vi "Get Exported Frames.vi"(8 "error in (no error)":errorcluster, 10 "GUID":string, 11 "Item Ref in":T4 format="%.0x") -> (0 "error out":errorcluster, 2 "Section":T1 {"Frames"."Signals"."Byte Order" items=["Little Endian", "Big Endian"]; "Frames"."Signals"."Data Type" items=["Signed", "Unsigned", "IEEE Float"]}, 3 "Section Ref out":T4 format="%.0x")   [LabVIEW 2015, in "Diagnostics Addon System Explorer.lvlib"]
uses:
  Diagnostics Addon System Explorer.lvlib
  <vilib>/NI Veristand/Custom Device Tools/Custom Device Utility Library/Custom Device Utility Library.lvlib
  <vilib>/NI Veristand/Custom Device Tools/Custom Device Utility Library/NI VeriStand - Search for Item by GUID.vi
  <vilib>/NI Veristand/Custom Device API/Custom Device API.lvlib
  Shared/Signal Parameters.ctl
  Shared/Diagnostics Addon Shared.lvlib
  Shared/Frame Parameters.ctl
  Shared/Exported Frames Cluster.ctl
  Shared/FG Action.ctl
  <vilib>/NI Veristand/Custom Device API/Custom Device Item Ref.ctl
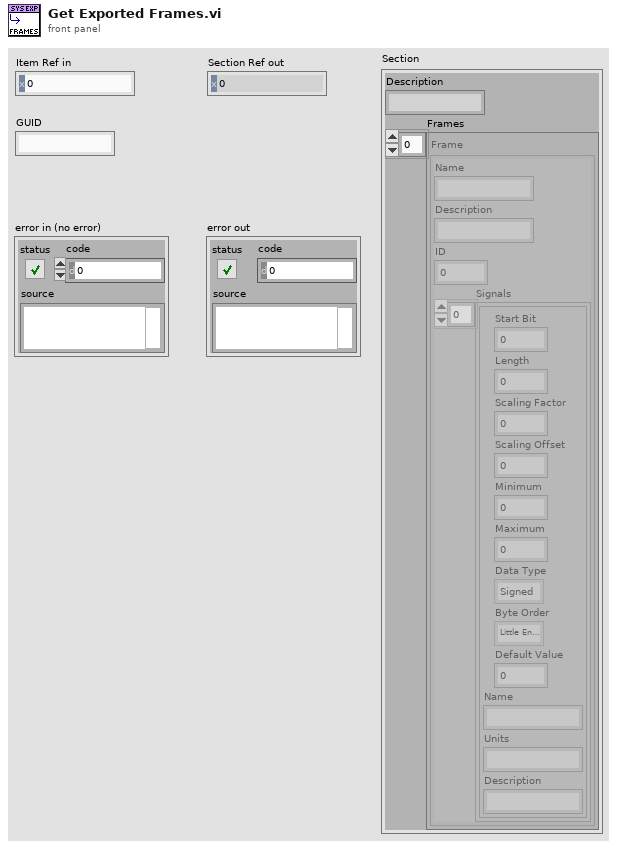
[diagram p1: front panel]
types:
  T1 = typedef "Diagnostics Addon System Explorer.lvlib/Exported Frames Cluster.ctl" = cluster{"Description":string, "Frames":T2[]}
  T2 = typedef "Diagnostics Addon Shared.lvlib/Frame Parameters.ctl" = cluster{"Name":string, "Description":string, "ID":u16, "Signals":T3[]}
  T3 = typedef "Diagnostics Addon Shared.lvlib/Signal Parameters.ctl" = cluster{"Start Bit":u8, "Length":u8, "Scaling Factor":dbl, "Scaling Offset":dbl, "Minimum":dbl, "Maximum":dbl, "Data Type":u32, "Byte Order":u32, "Default Value":dbl, "Name":string, "Units":string, "Description":string}
  T4 = typedef "Custom Device API.lvlib/Custom Device Item Ref.ctl" = u64
  T5 = typedef "Diagnostics Addon System Explorer.lvlib/FG Action.ctl" = enum16{"Get", "Set"}
  T6 = typedef "Custom Device API.lvlib/Custom Device Item Info.ctl" = cluster{"Name":string, "Is Channel":bool, "GUID":string, "Is Waveform":bool}
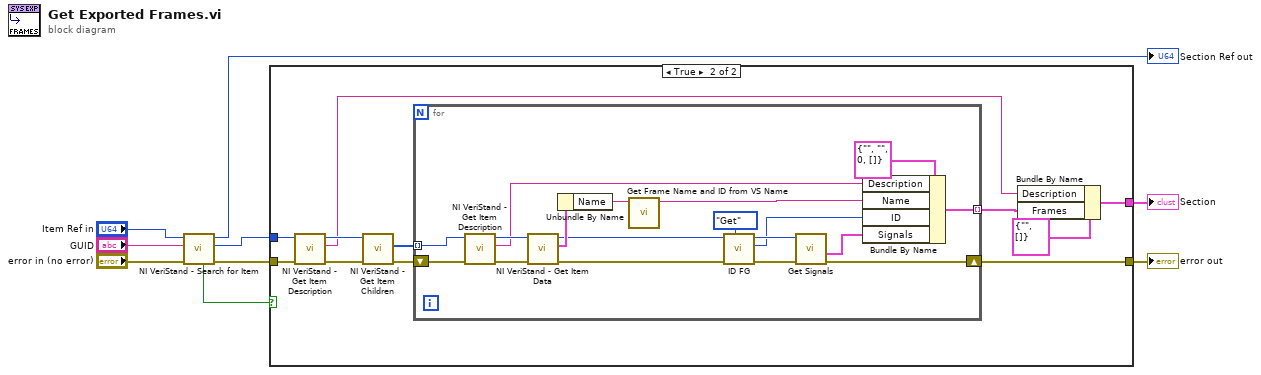
[diagram p0: block diagram]
diagram:
  n1 = call-poly <vilib>:"NI VeriStand - Search for Item.vi"("error in"="error in (no error)", "Item GUID"="GUID", "Section Ref in"="Item Ref in") -> ("error out"=w4:errorcluster, "Item Ref"=w3:T4, "Section Ref out"=→"Section Ref out":T4, "Found"=w2:bool)  [unwired: 5 in]
  n2 = case shown="True" w2 {
    tunnel: [_ w12] -> w1
    tunnel: [w10 w21] -> w5
    tunnel: w4 -> [w10 w16]
    tunnel: w3 -> [_ w18]
    frame False {
    }
    frame True {
      n3 = call <vilib>:"NI VeriStand - Get Item Description.vi"("error in (no error)"=w16, "Item Ref in"=w18) -> ("error out"=w15:errorcluster, "Description"=w13:string, "Item Ref out"=w17:T4)  [unwired: 7 out]
      n4 = call <vilib>:"NI VeriStand - Get Item Children.vi"("error in (no error)"=w15, "Item Ref in"=w17) -> ("error out"=w20:errorcluster, "Child Refs"=w19:T4[])  [unwired: 6 in, 2 out]
      n5 = for {
        tunnel: w19 -> [w36] mode=indexing
        shift-right: [w29] -> w21
        shift-left: w20 -> [w35]
        tunnel: [w25] -> w11 mode=indexing
        n6 = call <vilib>:"NI VeriStand - Get Item Description.vi"("error in (no error)"=w35, "Item Ref in"=w36) -> ("error out"=w38:errorcluster, "Description"=w34:string, "Item Ref out"=w39:T4)  [unwired: 7 out]
        n7 = call <vilib>:"NI VeriStand - Get Item Data.vi"("error in (no error)"=w38, "Item Ref in"=w39) -> ("error out"=w31:errorcluster, "Item Info"=w37:T6, "Item Ref out"=w30:T4)  [unwired: 7 out]
        n8 = Unbundle By Name(w37) -> ("Name"=w23:string)
        n9 = call "Get Frame Name and ID from VS Name.vi"("VS PID Name"=w23) -> ("PID Name"=w22:string)  [unwired: 9 in, 1 out]
        n10 = call "ID FG.vi"("Action"=FG_Action."Get", "error in (no error)"=w31, "Device Item Ref in"=w30) -> ("error out"=w32:errorcluster, "ID"=w27:u32, "Device Item Ref out"=w33:T4)  [unwired: 6 in]
        n11 = call "Get Signals.vi"("error in (no error)"=w32, "Device Item Ref out"=w33) -> ("error out"=w29:errorcluster, "Parameters"=w26:T3[])  [unwired: 6 in, 2 out]
        n12 = Bundle By Name(cluster=T2 {"Name"="", "Description"="", "ID"=0, "Signals"=[]}, "Description"=w34, "Name"=w22, "ID"=w27, "Signals"=w26) -> (w25:T2)
      }
      n13 = Bundle By Name(cluster=T1 {"Description"="", "Frames"=[]}, "Description"=w13, "Frames"=w11) -> (w12:T1)
    }
  }
  "error out" <- w5
  "Section" <- w1
